vi "ReadChans.vi"() -> ()   [LabVIEW 2017]
doc: "I. Description:\nThis example demonstrates how to make continuous, hardware-timed temperature measurement using a thermocouple.\n\nII. Instructions for Running:\n1. Specify the Physical Channel where you have connected the thermocouple.\n2. Enter the Minimum and Maximum temperature values in degrees C you expect to measure. A smaller range will allow a more accurate measurement.\n3. Enter the scan rate at which you want to run the acquisition.\n4. Specify the type of thermocouple you are using.\n5. Thermocouple measurements require cold-junction compensation (CJC) to correctly scale them. Specify the source of your cold-junction compensation.\n6. If your CJC source is \"Internal\", skip the rest of the steps.\n7. If your CJC source is \"Constant Value\", specify the value (usually room temperature) in degrees C.\n8. If your CJC source is \"Channel\", specify the CJC Channel name. \n9. Specify the appropriate Auto Zero Mode. See your device's hardware manual to find out if your device supports this attribute.\n\nIII. Block Diagram Steps:\n1. Create a Thermocouple (TC) temperature measurement channel.\n2. Get all the channels in the task.\n3. Convert channel(s) array to a comma-delimited channel string.\n4. This attribute is set to compensate for input offset errors. May not be supported by all devices*.\n5. Call the Timing VI to specify the hardware timing parameters. Use device's internal clock, continuous mode acquisition and the sample rate specified by the user.\n6. Call the Start VI to program and start the acquisition.\n7. Read N samples and plot it. By default, the Read VI reads all available samples, but you can specify how many samples to read at a time and the timeout value. Continue reading data until the stop button is pressed or an error occurs. \n8. Call the Clear Task VI to clear the Task.\n9. Use the popup dialog box to display an error if any.\n\n* If your device does not support Auto Zero Mode bypass Step 2, 3, and 4.\n\nIV. I/O Connections Overview:\nConnect your thermocouple to the terminals corresponding to the Physical Channel I/O Control value."
uses:
  <vilib>/Utility/error.llb/DialogType.ctl
  <vilib>/DAQmx/read.llb/DAQmx Read (Analog 1D Wfm NChan NSamp).vi
  <vilib>/Analysis/baseanly.llb/Mean (DBL).vi
  <vilib>/Waveform/WDTOps.llb/WDT Index Channel DBL.vi
  <vilib>/DAQmx/create/channels.llb/DAQmx Create Channel (AI-Voltage-Basic).vi
  <vilib>/DAQmx/configure/timing.llb/DAQmx Timing (Sample Clock).vi
  <vilib>/DAQmx/miscellaneous.llb/DAQmx Fill In Error Info.vi
  <vilib>/Analysis/NI_AALBase.lvlib
  <vilib>/ptbypt/NI_PtbyPt.lvlib
  <vilib>/Utility/miscctls.llb/LVRowAndColumnTypeDef.ctl
panel:
  out "AI Producer Iterations":i32
  in  "HW Channel":string="PXI1Slot3/ai0"
  out "Sample Rate (Hz)":string
  in  "Operator's Initials":string="IPS"
  in  "Test Cell":string(combo)="TC2"
  in  "Calibration Source":string(combo)="Line Driver"
  out "Channel Assignments":string[][](array[string])
  in  "error in 2":errorcluster
  in  "Data Tag":dbl=99.0 format="%.2p"
  out "Load Cell Min Peak":dbl format="%0.3f"
  out "Load Cell Max Peak":dbl format="%0.3f"
  in  "Stop":bool
  in  "Color Box":u32(colorbox)=16448250
  out "Results":i32[](listbox)=[0, 1]
  in  "num_chans":i32=8
  out "AI Consumer Iterations":i32=103
  in  "Logger Path":path=path "D:/LabView Data"
  out "Recorded Blocks":dbl=103.0
  in  "Force Record":bool caption="Force Record Enable"
  out "data 2":waveform(dbl)[](array[waveform])=[{"t0"=timestamp(3691443174.1812134 s since 1904-01-01), "dt"=0.1, "Y"=[0.06011962890625, 0.060577392578125], "attributes"=variant("NI_ChannelName"=variant(string "Dev2/ai0"), "NI_UnitDescription"=variant(string "Volts"))}, {"t0"=timestamp(3691443174.1812134 s since 1904-01-01), "dt"=0.1, "Y"=[-3.772430419921875, -3.772430419921875], "attributes"=variant("NI_ChannelName"=variant(string "Dev2/ai1"), "NI_UnitDescription"=variant(string "Volts"))}, {"t0"=timestamp(3691443174.1812134 s since 1904-01-01), "dt"=0.1, "Y"=[-3.286895751953125, -3.286590576171875], "attributes"=variant("NI_ChannelName"=variant(string "Dev2/ai2"), "NI_UnitDescription"=variant(string "Volts"))}, {"t0"=timestamp(3691443174.1812134 s since 1904-01-01), "dt"=0.1, "Y"=[-5.0, -5.0], "attributes"=variant("NI_ChannelName"=variant(string "Dev2/ai3"), "NI_UnitDescription"=variant(string "Volts"))}, {"t0"=timestamp(3691443174.1812134 s since 1904-01-01), "dt"=0.1, "Y"=[-2.80426025390625, -2.80426025390625], "attributes"=variant("NI_ChannelName"=variant(string "Dev2/ai4"), "NI_UnitDescription"=variant(string "Volts"))}, {"t0"=timestamp(3691443174.1812134 s since 1904-01-01), "dt"=0.1, "Y"=[-5.0, -5.0], "attributes"=variant("NI_ChannelName"=variant(string "Dev2/ai5"), "NI_UnitDescription"=variant(string "Volts"))}, {"t0"=timestamp(3691443174.1812134 s since 1904-01-01), "dt"=0.1, "Y"=[0.137481689453125, 0.13763427734375], "attributes"=variant("NI_ChannelName"=variant(string "Dev2/ai6"), "NI_UnitDescription"=variant(string "Volts"))}, {"t0"=timestamp(3691443174.1812134 s since 1904-01-01), "dt"=0.1, "Y"=[-4.823455810546875, -4.823455810546875], "attributes"=variant("NI_ChannelName"=variant(string "Dev2/ai7"), "NI_UnitDescription"=variant(string "Volts"))}]
  out "Waveform Chart":waveform(dbl)[](graph)=[{"t0"=timestamp(3691443174.1812134 s since 1904-01-01), "dt"=0.2, "Y"=[0.0603485107421875], "attributes"=variant("NI_ChannelName"=variant(string "AI0"), "NI_UnitDescription"=variant(string "V"))}, {"t0"=timestamp(3691443174.1812134 s since 1904-01-01), "dt"=0.2, "Y"=[-3.772430419921875], "attributes"=variant("NI_ChannelName"=variant(string "AI1"), "NI_UnitDescription"=variant(string "V"))}, {"t0"=timestamp(3691443174.1812134 s since 1904-01-01), "dt"=0.2, "Y"=[-3.2867431640625], "attributes"=variant("NI_ChannelName"=variant(string "AI2"), "NI_UnitDescription"=variant(string "V"))}, {"t0"=timestamp(3691443174.1812134 s since 1904-01-01), "dt"=0.2, "Y"=[-5.0], "attributes"=variant("NI_ChannelName"=variant(string "AI3"), "NI_UnitDescription"=variant(string "V"))}, {"t0"=timestamp(3691443174.1812134 s since 1904-01-01), "dt"=0.2, "Y"=[-2.80426025390625], "attributes"=variant("NI_ChannelName"=variant(string "AI4"), "NI_UnitDescription"=variant(string "V"))}, {"t0"=timestamp(3691443174.1812134 s since 1904-01-01), "dt"=0.2, "Y"=[-5.0], "attributes"=variant("NI_ChannelName"=variant(string "AI5"), "NI_UnitDescription"=variant(string "V"))}, {"t0"=timestamp(3691443174.1812134 s since 1904-01-01), "dt"=0.2, "Y"=[0.1375579833984375], "attributes"=variant("NI_ChannelName"=variant(string "AI6"), "NI_UnitDescription"=variant(string "V"))}, {"t0"=timestamp(3691443174.1812134 s since 1904-01-01), "dt"=0.2, "Y"=[-4.823455810546875], "attributes"=variant("NI_ChannelName"=variant(string "AI7"), "NI_UnitDescription"=variant(string "V"))}]
  in  "Run Letter":string="a"
  out "Recording":bool
  in  "Num_Blocks":dbl=100.0
  in  "Rate":dbl=10.0 format="%0.2f"
  # "Directions:\n1) Use the Excel spreadsheet \"Labview Chan Map Cal.xlsm\" to edit the channel names, device assignments, units, and scaling.\n2) Press the \"Save ChnCfg.txt\" button on the spreadshseet to export the parameters from step 1) to a \"ChnCfg.txt\" file within the /Constants folder.\n3)  Use the Druck Genii DPI612 to apply a calibration voltage to each PXI-6143 analog input.  Verify that all voltages match calibration voltage to ±.001 V."
  # "For instructions, select Help>>Show Context Help"
  # "Timing Parameters"
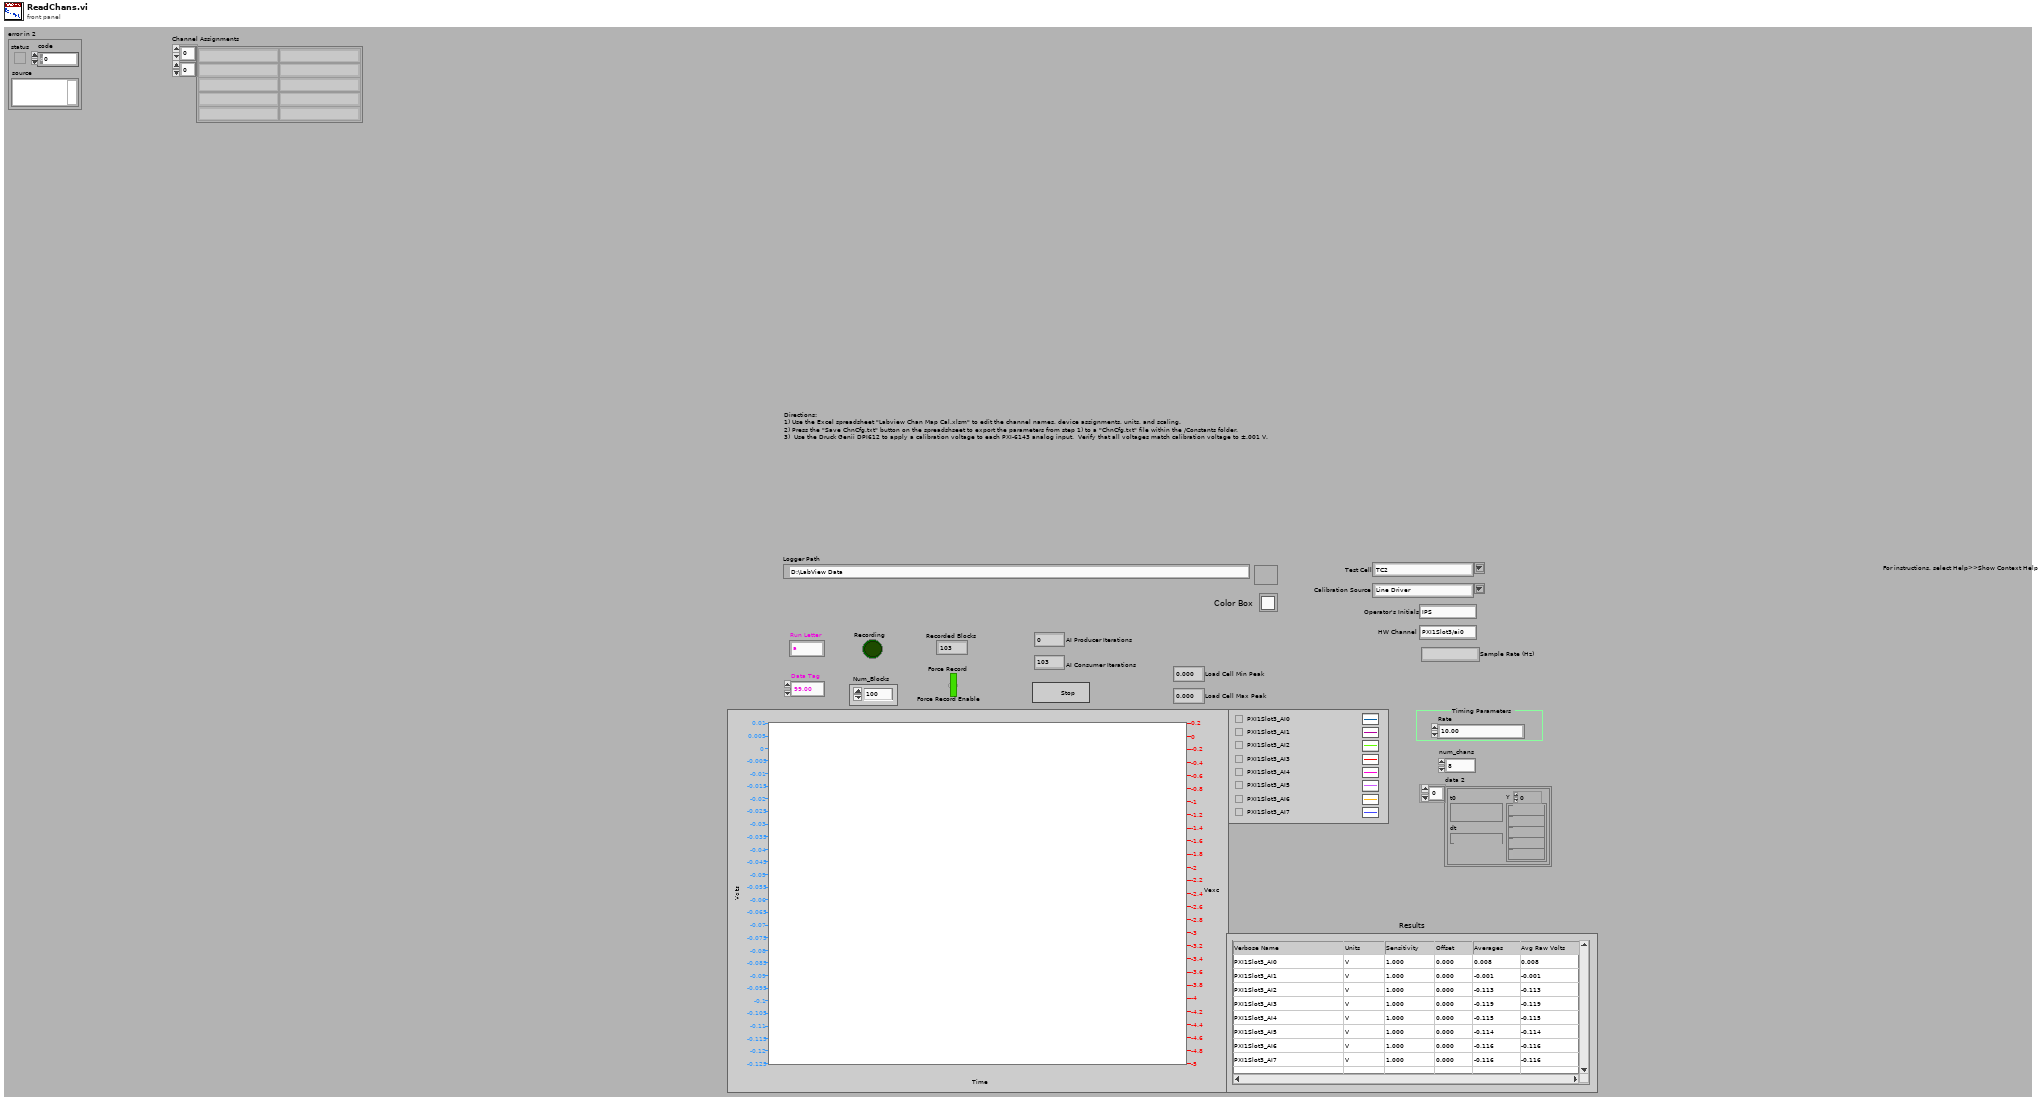
[diagram p1: front panel]
types:
  T1 = cluster{"Test Cell":string, "Calibration Source":string, "Operator's Initials":string, "HW Channel":string, "Sample Rate (Hz)":string}
  T2 = typedef "DialogType.ctl" = u16
  T3 = typedef "LVRowAndColumnTypeDef.ctl" = cluster{"Row":i32, "Column":i32}
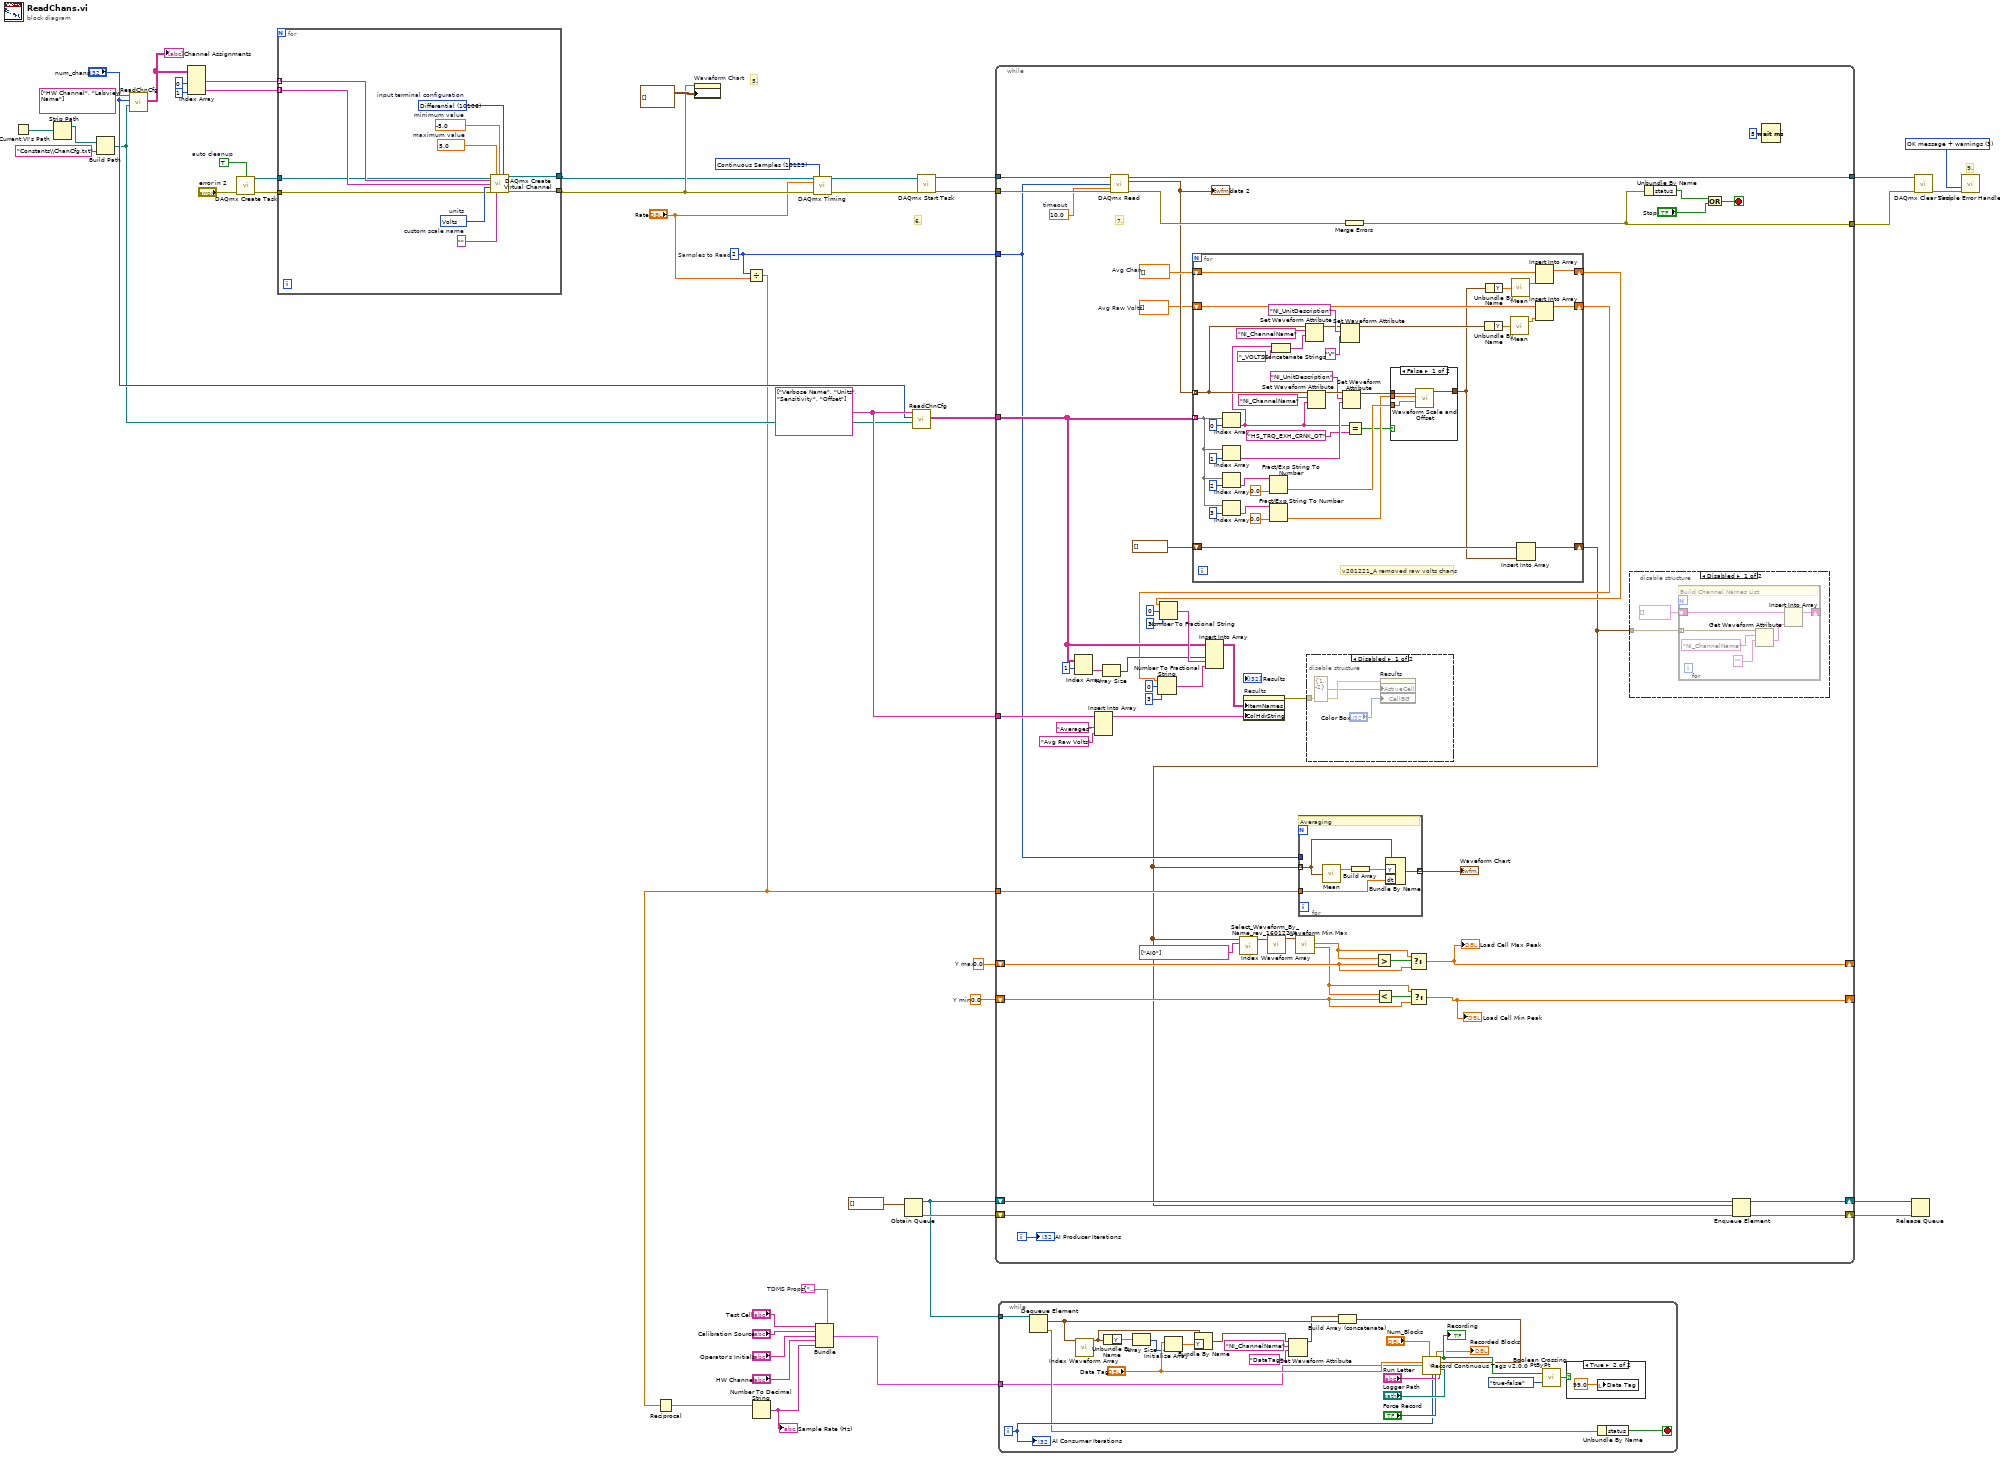
[diagram p0: block diagram]
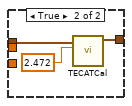
[diagram p5: hidden frame]
diagram:
  w9 = T1 {"Test Cell"="TC2", "Calibration Source"="Line Driver", "Operator's Initials"="IPS", "HW Channel"="PXI1Slot3/ai0", "Sample Rate (Hz)"=""}  # TDMS Props
  w26 = TRUE  # auto cleanup
  w34 = string[] ["Verbose Name", "Units", "Sensitivity", "Offset"] ("Search Strings")
  w30 = 0.0  # Y min
  w31 = 0.0  # Y max
  w29 = 2 ("number of samples per channel")
  w42 = T2 3 items=["no dialog", "OK message", "continue or stop message", "OK message + warnings", "continue/stop + warnings"] ("type of dialog (OK msg:1)")
  w35 = 10123 items=["Finite Samples"=10178, "Continuous Samples"=10123] ("sample mode")
  # "Samples to Read"
  # "9."
  # "5."
  # "6."
  n1 = Current VI's Path() -> (path=w12:path)
  n2 = Strip Path(path=w12) -> (stripped path=w11:path)  [unwired: 1 out]
  n3 = Build Path(base path=w11, name or relative path="Constants\\ChanCfg.txt") -> (appended path=w13:path)
  n4 = call "ReadChnCfg.vi"("file path (uses default if empty)"=w13, "num_chans"="num_chans", "Search Strings"=string[] ["HW Channel", "Labview Name"]) -> ("Table Minus Headers"=w24:string[][])  [unwired: 4 in, 4 out]
  "Channel Assignments" <- w24
  n5 = Index Array(array=w24, index (col) #1=0 ("disabled index (col)"), index (col) #2=1 ("index (col)")) -> (element #1=w19:string[], element #2=w18:string[])  [unwired: 2 in]
  n6 = call <vilib>:"DAQmx Create Task.vi"("auto cleanup"=w26, "error in"="error in 2") -> ("task out"=w21:refnum<k21>, "error out"=w20:errorcluster)  [unwired: 12 in]
  n7 = for {
    tunnel: [w53] -> w16
    tunnel: [w52] -> w17
    tunnel: w21 -> [w49]
    tunnel: w20 -> [w48]
    tunnel: w19 -> [w51] mode=indexing
    tunnel: w18 -> [w50] mode=indexing
    w54 = 10106 items=["default"=-1, "RSE"=10083, "NRSE"=10078, "Differential"=10106, "Pseudodifferential"=12529]  # input terminal configuration
    w55 = 10348 items=["Volts"=10348, "From Custom Scale"=10065]  # units
    w56 = ""  # custom scale name
    w57 = -5.0  # minimum value
    w58 = 5.0  # maximum value
    n8 = call-poly <vilib>:"DAQmx Create Virtual Channel.vi"("task in"=w49, "maximum value"=w58, "minimum value"=w57, "input terminal configuration"=w54, "physical channels"=w51, "name to assign"=w50, "units"=w55, "error in"=w48, "custom scale name"=w56) -> ("task out"=w53:refnum<k21>, "error out"=w52:errorcluster)  [unwired: 5 in]
  }
  n9 = property on="Waveform Chart" class="WFChart (strict)"(error in=w17, "History Data"=waveform(dbl)[][] []) -> ()  [unwired: 1 in, 2 out]
  n10 = Divide(x=w29, y="Rate") -> (x/y=w2:dbl)
  n11 = Reciprocal(x=w2) -> (1/x=w1:dbl)
  n12 = Number To Decimal String(number=w1) -> (decimal integer string=w4:string)  [unwired: 1 in]
  "Sample Rate (Hz)" <- w4
  n13 = call-poly <vilib>:"DAQmx Timing.vi"("task/channels in"=w16, "sample mode"=w35, "rate"="Rate", "error in"=w17) -> ("task out"=w43:refnum<k21>, "error out"=w32:errorcluster)  [unwired: 10 in]
  n14 = Bundle(cluster=w9, "Test Cell"="Test Cell", "Calibration Source"="Calibration Source", "Operator's Initials"="Operator's Initials", "HW Channel"="HW Channel", "Sample Rate (Hz)"=w4) -> (w3:T1)
  n15 = Obtain Queue(element data type=waveform(dbl)[] [] ("appended array")) -> (queue out=w36:refnum<queue>, error out=w39:errorcluster)  [unwired: 4 in, 1 out]
  n16 = call "ReadChnCfg.vi"("file path (uses default if empty)"=w13, "num_chans"="num_chans", "Search Strings"=w34) -> ("Table Minus Headers"=w28:string[][])  [unwired: 4 in, 4 out]
  n17 = call <vilib>:"DAQmx Start Task.vi"("task/channels in"=w43, "error in"=w32) -> ("task out"=w45:refnum<k21>, "error out"=w46:errorcluster)  [unwired: 12 in]
  n18 = while {
    tunnel: w45 -> [w110]
    tunnel: w46 -> [w109]
    tunnel: [w108] -> w44
    tunnel: w29 -> [w69]
    shift-right: [w101] -> w38
    shift-left: w36 -> [w103]
    shift-right: [w100] -> w37
    shift-left: w39 -> [w102]
    tunnel: [w85] -> w33
    tunnel: w28 -> [w88]
    tunnel: w34 -> [w97]
    shift-right: [w74] -> _
    shift-left: w31 -> [w75]
    shift-right: [w71] -> _
    shift-left: w30 -> [w70]
    tunnel: w2 -> [w68]
    i -> [w59]
    stop <- w105 stop-if-true
    w67 = dbl[] []  # Avg Raw Volts
    w99 = dbl[] []  # Avg Chan
    w106 = 10.0  # timeout
    # "7."
    n19 = Index Array(array=w88, index (row)=1) -> (element=w91:string[])  [unwired: 1 in]
    n20 = Insert Into Array(array=w97, new element #1="Averages" ("new element/subarray"), new element #2="Avg Raw Volts" ("new element/subarray")) -> (w89:string[])  [unwired: 1 in]
    n21 = Array Size(array=w91) -> (size(s)=w63:i32)
    n22 = call-poly <vilib>:"DAQmx Read.vi"("task/channels in"=w110, "number of samples per channel"=w69, "timeout"=w106, "error in"=w109) -> ("task out"=w108:refnum<k21>, "data"=w82:waveform(dbl)[], "error out"=w86:errorcluster)  [unwired: 9 in]
    "data 2" <- w82
    n23 = for {
      tunnel: w82 -> [w140] mode=indexing
      shift-right: [w159] -> w83
      shift-left: w99 -> [w158]
      tunnel: w88 -> [w150] mode=indexing
      shift-right: [w156] -> w60
      shift-left: waveform(dbl)[] [] -> [w157]
      shift-right: [w132] -> w62
      shift-left: w67 -> [w134]
      # "v201221_A removed raw volts chans"
      n24 = Index Array(array=w150, index=0) -> (element=w129:string)
      n25 = Index Array(array=w150, index=1) -> (element=w153:string)
      n26 = Index Array(array=w150, index=2) -> (element=w149:string)
      n27 = Index Array(array=w150, index=3) -> (element=w145:string)
      n28 = Fract/Exp String To Number(string=w149, default (0 dbl)=0.0) -> (number=w147:dbl)  [unwired: 2 in, 1 out]
      n29 = Fract/Exp String To Number(string=w145, default (0 dbl)=0.0) -> (number=w144:dbl)  [unwired: 2 in, 1 out]
      n30 = Concatenate Strings(w129, "_VOLTS" ("string")) -> (w139:string)
      n31 = Set Waveform Attribute(5:w139, 6:"NI_ChannelName" ("name"), 7:w140) -> (3:w142:waveform(dbl))  [unwired: 1 in, 2 out]
      n32 = Set Waveform Attribute(5:w129, 6:"NI_ChannelName" ("name"), 7:w140) -> (3:w163:waveform(dbl))  [unwired: 1 in, 2 out]
      n33 = Set Waveform Attribute(5:"V" ("string"), 6:"NI_UnitDescription" ("name"), 7:w142) -> (3:w131:waveform(dbl))  [unwired: 1 in, 2 out]
      n34 = Set Waveform Attribute(5:w153, 6:"NI_UnitDescription" ("name"), 7:w163) -> (3:w161:waveform(dbl))  [unwired: 1 in, 2 out]
      n35 = Equal?(x=w129, y="HS_TRQ_EXH_CRNK_OT" ("String")) -> (x = y?=w128:bool)
      n36 = case shown="False" w128 {
        tunnel: w161 -> [w168 w170]
        tunnel: w147 -> [w167 _]
        tunnel: w144 -> [w166 _]
        tunnel: [w165 w171] -> w127
        frame False {
          n37 = call <vilib>:"Waveform Scale and Offset.vi"("scale"=w167, "offset"=w166, "waveform in"=w168) -> ("waveform out"=w165:waveform(dbl))  [unwired: 7 in, 1 out]
        }
        frame True {
          n38 = call "TECATCal.vi"("dZeroLvl"=2.472, "wfmIN"=w170) -> ("wfmOUT"=w171:waveform(dbl))  [unwired: 9 in]
        }
      }
      n39 = Unbundle By Name(w131) -> ("Y"=w136:dbl[])
      n40 = Unbundle By Name(w127) -> ("Y"=w160:dbl[])
      n41 = call-poly <vilib>:"Mean.vi"("X"=w136) -> ("mean"=w133:dbl)  [unwired: 1 out]
      n42 = call-poly <vilib>:"Mean.vi"("X"=w160) -> ("mean"=w135:dbl)  [unwired: 1 out]
      n43 = Insert Into Array(array=w157, new element=w127) -> (w156:waveform(dbl)[])  [unwired: 1 in]
      n44 = Insert Into Array(array=w158, new element=w135) -> (w159:dbl[])  [unwired: 1 in]
      n45 = Insert Into Array(array=w134, new element=w133) -> (w132:dbl[])  [unwired: 1 in]
    }
    n46 = Number To Fractional String(number=w62, width (-)=i16 0, precision (6)=i16 3) -> (F-format string=w61:string[])  [unwired: 1 in]
    n47 = Number To Fractional String(number=w83, width (-)=i16 0, precision (6)=i16 3) -> (F-format string=w93:string[])  [unwired: 1 in]
    n48 = Insert Into Array(array=w88, index (col)=w63, new element #1=w93, new element #2=w61) -> (w90:string[][])  [unwired: 1 in]
    n49 = call "Select_Waveform_By_Name_rev_160122_A.vi"("Array"=string[] ["AI0"], "Waveform Array"=w60) -> ("Array 2"=w79:waveform(dbl)[])  [unwired: 9 in]
    n50 = property on="Results" class="MCListbox (strict)"("ItemNames"=w90, "ColHdrString"=w89) -> (error out=w87:errorcluster)  [unwired: 2 in, 1 out]
    n51 = call-poly <vilib>:"Index Waveform Array.vi"("waveform array"=w79) -> ("waveform"=w78:waveform(dbl))  [unwired: 9 in, 1 out]
    n52 = call <vilib>:"Waveform Min Max.vi"("waveform in"=w78) -> ("Y min"=w72:dbl, "Y max"=w76:dbl)  [unwired: 5 in, 4 out]
    n53 = for {
      tunnel: w60 -> [w125] mode=indexing
      tunnel: [w126] -> w81 mode=indexing
      tunnel: w69 -> [_]
      tunnel: w68 -> [w122]
      # "Averaging"
      n54 = call-poly <vilib>:"Mean.vi"("X"=w125) -> ("mean"=w124:dbl)  [unwired: 1 out]
      n55 = Build Array(w124) -> (w123:dbl[])
      n56 = Bundle By Name(cluster=w125, "Y"=w123, "dt"=w122) -> (w126:waveform(dbl))
    }
    "Waveform Chart" <- w81
    n57 = disable-structure shown="Disabled" {
      disable-tunnel: w87 -> [w121 _]
      frame Disabled {
        n58 = property on="Results" class="MCListbox (strict)"(error in=w121, "ActiveCell"=T3 {"Row"=1, "Column"=-2} ("Active Cell:Active Cell"), "CellBG"="Color Box") -> ()  [unwired: 1 in, 2 out]
      }
      frame Enabled {
      }
    }
    n59 = Merge Errors(w86) -> (w85:errorcluster)
    n60 = Greater?(x=w76, y=w75) -> (0:w77:bool)
    n61 = Less?(x=w72, y=w70) -> (x < y?=w73:bool)
    n62 = Select(t=w76, s=w77, f=w75) -> (s? t:f=w74:dbl)
    "Load Cell Max Peak" <- w74
    n63 = Select(t=w72, s=w73, f=w70) -> (s? t:f=w71:dbl)
    "Load Cell Min Peak" <- w71
    n64 = disable-structure shown="Disabled" {
      disable-tunnel: w60 -> [w111 _]
      frame Disabled {
        n65 = for {
          tunnel: w111 -> [w117] mode=indexing
          shift-right: [w113] -> _
          shift-left: string[] [] ("Array") -> [w118]
          # "Build Channel Names List"
          n66 = Get Waveform Attribute(5:"" ("name"), 6:"NI_ChannelName" ("name"), 7:w117) -> (1:w114:string)  [unwired: 1 in, 3 out]
          n67 = Insert Into Array(array=w118, new element=w114) -> (w113:string[])  [unwired: 1 in]
        }
      }
      frame Enabled {
      }
    }
    n68 = Unbundle By Name(w85) -> ("status"=w107:bool)
    n69 = Or(x=w107, y="Stop") -> (x .or. y?=w105:bool)
    n70 = Enqueue Element(queue=w103, element=w60, error in (no error)=w102) -> (queue out=w101:refnum<queue>, error out=w100:errorcluster)  [unwired: 1 in, 1 out]
    n71 = Wait (ms)(milliseconds to wait=u32 5) -> ()  [unwired: 1 out]
    "AI Producer Iterations" <- w59
  }
  n72 = while {
    tunnel: w36 -> [w187]
    tunnel: w3 -> [w172]
    i -> [w186]
    stop <- w184 stop-if-true
    n73 = Dequeue Element(queue=w187) -> (element=w175:waveform(dbl)[], error out=w185:errorcluster)  [unwired: 2 in, 2 out]
    n74 = call-poly <vilib>:"Index Waveform Array.vi"("waveform array"=w175) -> ("waveform"=w179:waveform(dbl))  [unwired: 9 in, 1 out]
    n75 = Unbundle By Name(w179) -> ("Y"=w183:dbl[])
    n76 = Array Size(array=w183) -> (size(s)=w181:i32)
    n77 = Initialize Array("Data Tag", w181) -> (w180:dbl[])
    n78 = Bundle By Name(cluster=w179, "Y"=w180) -> (w178:waveform(dbl))
    n79 = Set Waveform Attribute(5:"DataTag" ("name"), 6:"NI_ChannelName" ("name"), 7:w178) -> (3:w174:waveform(dbl))  [unwired: 1 in, 2 out]
    n80 = Build Array (concatenate)(w174, w175) -> (w173:waveform(dbl)[])
    n81 = call "Record Continuous Tags v2.0.0.vi"("Num_Blocks"="Num_Blocks", "Data Tag"="Data Tag", "Waveform Array In"=w173, "TDMS Props"=w172, "path"="Logger Path", "Main Count"=w186, "Force Record"="Force Record", "Run Letter"="Run Letter") -> ("Recorded Blocks"=→"Recorded Blocks":dbl, "Record Cmd"=w193:bool)  [unwired: 5 in, 1 out]
    "Recording" <- w193
    n82 = call <vilib>:"Boolean Crossing PtByPt.vi"("direction"=enum16{"either", "false-true", "true-false"}."true-false", "input"=w193) -> ("crossing"=w194:bool)  [unwired: 1 in]
    n83 = case shown="True" w194 {
      frame False {
      }
      frame True {
        n84 = local write "Data Tag"(99.0 ("y")) -> ()
      }
    }
    n85 = Unbundle By Name(w185) -> ("status"=w184:bool)
    "AI Consumer Iterations" <- w186
  }
  n86 = Release Queue(queue=w38, error in (no error)=w37) -> ()  [unwired: 1 in, 3 out]
  n87 = call <vilib>:"DAQmx Clear Task.vi"("task in"=w44, "error in"=w33) -> ("error out"=w47:errorcluster)  [unwired: 13 in]
  n88 = call <vilib>:"Simple Error Handler.vi"("type of dialog (OK msg:1)"=w42, "error in (no error)"=w47) -> ()  [unwired: 3 in, 5 out]
